vi "LoadDev.vi"() -> (0 "ViStatus":T2, 1 "ModuleInfo":T4 {"DacScaleCoef" format="%#_2g"; "DacOffsetCoef" format="%#_2g"}, 3 "InterfaceInfo":T3)   [LabVIEW 2010]
panel:
  in  "step":T1(tab)
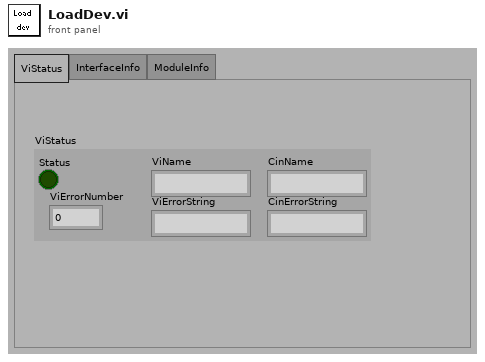
[diagram p1: front panel]
types:
  T1 = enum32{"ViStatus", "InterfaceInfo", "ModuleInfo"}
  T2 = cluster{"Status":bool, "ViErrorNumber":u32, "ViName":string, "ViErrorString":string, "CinName":string, "CinErrorString":string}
  T3 = cluster{"DllVersion":u32, "InterfaceType":u32, "InterfaceInstance":u32, "ModuleHandle":u32, "ReadBuffersParsArray":cluster{"Buffer":i16[], "ReadOv":u32, "ReadEvent":u32}[], "WriteBuffersParsArray":cluster{"Buffer":i16[], "WriteOv":u32, "WriteEvent":u32}[]}
  T4 = cluster{"VirtualSlot":u16, "ModuleName":string, "SerialNumber":string, "UsbSpeed":u8, "AvrVersion":string, "ModuleRevision":string, "DspType":string, "IsDacPresented":bool, "DspLoading":bool, "DspVersion":string, "DspClockout":u32, "AdcOffsetCoef":sgl[], "AdcScaleCoef":sgl[], "DacOffsetCoef":sgl[], "DacScaleCoef":sgl[]}
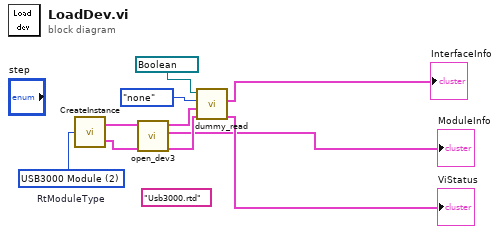
[diagram p0: block diagram]
diagram:
  w10 = u32 2 items=["Unknown Module", "USB2185 Module", "USB3000 Module"]  # RtModuleType
  (unwired) "Usb3000.rtd" ("DspDriverFile")
  n1 = call "CreateInstance.vi"("InterfaceType"=w10) -> ("InterfaceInfo"=w7:T3, "ViStatus"=w8:T2)
  n2 = call "open_dev3.vi"("ViStatus"=w8, "InterfaceInfo 2"=w7) -> ("ViStatus 2"=w5:T2, "ModuleInfo"=→"ModuleInfo":T4, "InterfaceInfo"=w6:T3)  [unwired: 2 in, 1 out]
  n3 = call "dummy_read.vi"("ViStatusOut 2"=w5, "InterfaceInfoOut 2"=w6, "SyncType3000"=enum16{"none", "TTL", "TTL_kadr", "analog"}."none", "Ctrl Reference"=refnum<vi> refnum) -> ("ViStatusOut"=→"ViStatus":T2, "InterfaceInfoOut"=→"InterfaceInfo":T3)  [unwired: 2 in]
